vi "tdm.vi"() -> ()   [LabVIEW 2016]
panel:
  out "Waveform Graph":dynamicdata(graph)
  in  "add":dbl(slide) scale=0.0..10.0
  in  "multiplier":dbl(slide) scale=-5.0..5.0
  out "Sine 3":dynamicdata(graph) caption="Sine"
  out "Sine 2":dynamicdata(graph) caption="Sine"
  out "Sine":dynamicdata(graph)
  in  "Tri freq 3":dbl(slide)=10.1 caption="Frequency" scale=0.0..500.0
  in  "tri Amp 3":dbl(slide)=1.0 caption="Amplitude" scale=0.0..10.0
  in  "SQ freq 2":dbl(slide)=10.1 caption="Frequency" scale=0.0..50.0
  in  "Sq Amp 2":dbl(slide)=1.0 caption="Amplitude" scale=0.0..10.0
  in  "Sine freq":dbl(slide)=10.1 caption="Frequency" scale=0.0..100.0
  in  "Sine Amp":dbl(slide)=1.0 caption="Amplitude" scale=0.0..10.0
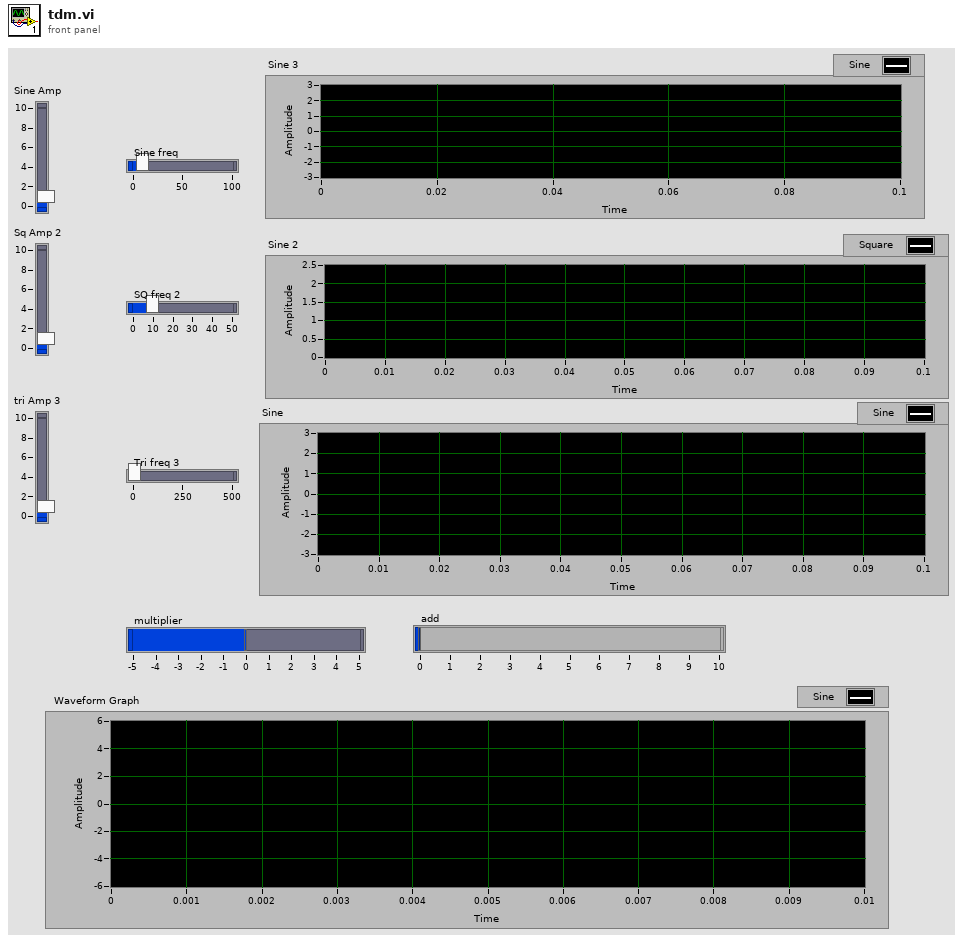
[diagram p1: front panel]
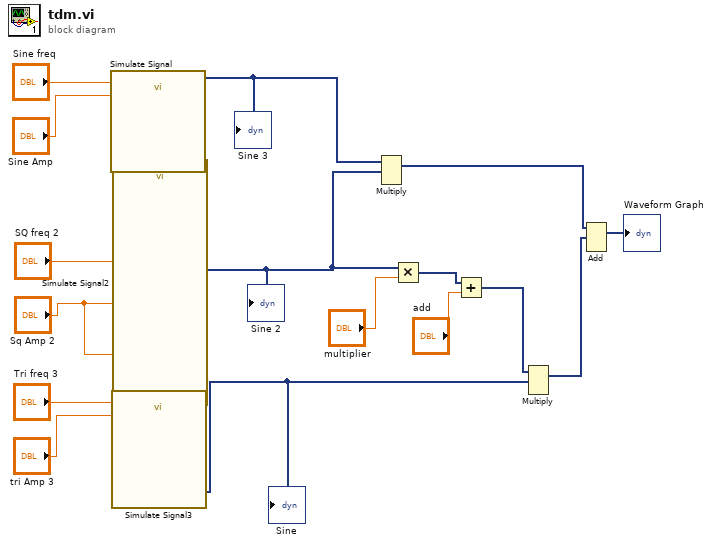
[diagram p0: block diagram]
diagram:
  n1 = call "Simulate Signal"("Frequency"="Sine freq", "Amplitude"="Sine Amp") -> ("Sine"=w3:dynamicdata)  [unwired: 12 in, 1 out]
  "Sine 3" <- w3
  n2 = call "Simulate Signal3"("Frequency"="Tri freq 3", "Amplitude"="tri Amp 3") -> ("Sine"=w2:dynamicdata)  [unwired: 12 in, 1 out]
  "Sine" <- w2
  n3 = call "Simulate Signal2"("Offset"="Sq Amp 2", "Frequency"="SQ freq 2", "Amplitude"="Sq Amp 2") -> ("Square"=w9:dynamicdata)  [unwired: 11 in, 1 out]
  "Sine 2" <- w9
  n4 = Multiply(1:w9, 2:w3) -> (0:w7:dynamicdata)  [unwired: 1 in, 1 out]
  n5 = Multiply(x=w9, y="multiplier") -> (x*y=w11:dynamicdata)
  n6 = Add(x=w11, y="add") -> (x+y=w10:dynamicdata)
  n7 = Multiply(1:w2, 2:w10) -> (0:w8:dynamicdata)  [unwired: 1 in, 1 out]
  n8 = Add(1:w8, 2:w7) -> (0:→"Waveform Graph":dynamicdata)  [unwired: 1 in, 1 out]
